vi "FilePath.vi"(9 "Data Root Path":path, 10 "File Type":enum16{"Thru", "NEXT", "FEXT"}(ring), 11 "Product Type":enum16{"QSFP28", "SFP28", "MiniSAS"}(ring)) -> (2 "File Path List":path[](array[path]), 3 "FileName List (not suffix)":string[](array[string]))   [LabVIEW 2011]
uses:
  <vilib>/Utility/file.llb/Read From Spreadsheet File (string).vi
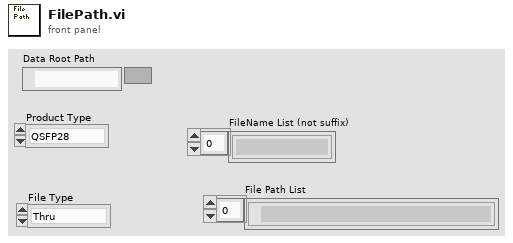
[diagram p1: front panel]
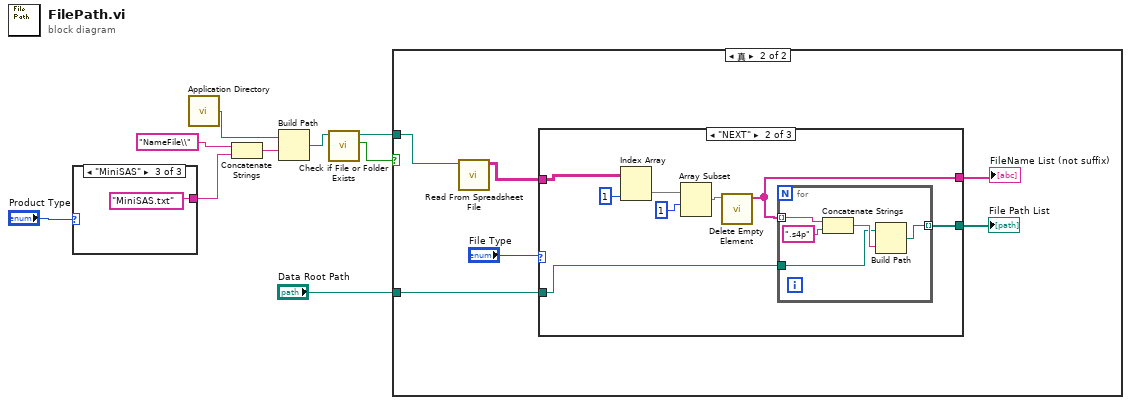
[diagram p0: block diagram]
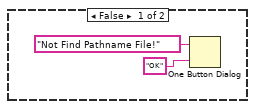
[diagram p2: hidden frame]
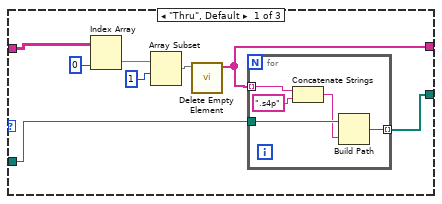
[diagram p3: hidden frame]
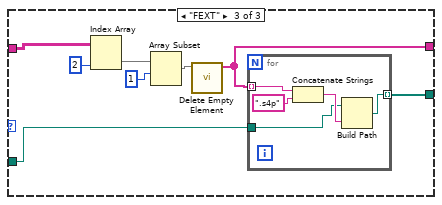
[diagram p4: hidden frame]
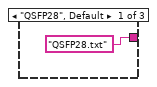
[diagram p5: hidden frame]
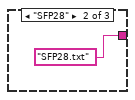
[diagram p6: hidden frame]
diagram:
  n1 = case shown="\"MiniSAS\"" "Product Type" {
    tunnel: ["QSFP28.txt" ("名称或相对路径") "SFP28.txt" ("名称或相对路径") "MiniSAS.txt" ("名称或相对路径")] -> w7
    frame "QSFP28", Default {
    }
    frame "SFP28" {
    }
    frame "MiniSAS" {
    }
  }
  n2 = call <vilib>:"Application Directory.vi"() -> ("Application Directory"=w8:path)
  n3 = Concatenate Strings("NameFile\\" ("字符串"), w7) -> (w5:string)
  n4 = Build Path(base path=w8, name or relative path=w5) -> (appended path=w4:path)
  n5 = call <vilib>:"Check if File or Folder Exists.vi"("path"=w4) -> ("file or folder exists?"=w2:bool, "dup path"=w3:path)  [unwired: 8 in, 1 out]
  n6 = case shown="真" w2 {
    tunnel: w3 -> [_ w17]
    tunnel: "Data Root Path" -> [_ w16]
    frame False {
      n7 = One Button Dialog(message="Not Find Pathname File!" ("消息"), button name ("OK")="OK" ("按钮名称（“确定”）")) -> ()  [unwired: 1 out]
    }
    frame True {
      n8 = call-poly <vilib>:"Read From Spreadsheet File.vi"("file path (dialog if empty)"=w17) -> ("all rows"=w19:string[][])  [unwired: 6 in, 4 out]
      n9 = case shown="\"NEXT\"" "File Type" {
        tunnel: w19 -> [w28 w41 w54]
        tunnel: [w23 w36 w49] -> w18
        tunnel: w16 -> [w22 w35 w48]
        tunnel: [w21 w34 w47] -> w15
        frame "Thru", Default {
          n10 = Index Array(array=w28, index (col)=0 ("禁用的索引 (列)")) -> (element=w26:string[])  [unwired: 1 in]
          n11 = Array Subset(array=w26, index=1 ("索引")) -> (w24:string[])  [unwired: 1 in]
          n12 = call "Delete Empty Element.vi"("input"=w24) -> ("output"=w23:string[])  [unwired: 10 in]
          n13 = for {
            tunnel: w23 -> [w33] mode=indexing
            tunnel: w22 -> [w31]
            tunnel: [w29] -> w21 mode=indexing
            n14 = Concatenate Strings(w33, ".s4p" ("字符串")) -> (w30:string)
            n15 = Build Path(base path=w31, name or relative path=w30) -> (appended path=w29:path)
          }
        }
        frame "NEXT" {
          n16 = Index Array(array=w41, index (col)=1 ("禁用的索引 (列)")) -> (element=w39:string[])  [unwired: 1 in]
          n17 = Array Subset(array=w39, index=1 ("索引")) -> (w37:string[])  [unwired: 1 in]
          n18 = call "Delete Empty Element.vi"("input"=w37) -> ("output"=w36:string[])  [unwired: 10 in]
          n19 = for {
            tunnel: w36 -> [w46] mode=indexing
            tunnel: w35 -> [w43]
            tunnel: [w42] -> w34 mode=indexing
            n20 = Concatenate Strings(w46, ".s4p" ("字符串")) -> (w44:string)
            n21 = Build Path(base path=w43, name or relative path=w44) -> (appended path=w42:path)
          }
        }
        frame "FEXT" {
          n22 = Index Array(array=w54, index (col)=2 ("禁用的索引 (列)")) -> (element=w52:string[])  [unwired: 1 in]
          n23 = Array Subset(array=w52, index=1 ("索引")) -> (w50:string[])  [unwired: 1 in]
          n24 = call "Delete Empty Element.vi"("input"=w50) -> ("output"=w49:string[])  [unwired: 10 in]
          n25 = for {
            tunnel: w49 -> [w59] mode=indexing
            tunnel: [w57] -> w47 mode=indexing
            tunnel: w48 -> [w55]
            n26 = Concatenate Strings(w59, ".s4p" ("字符串")) -> (w56:string)
            n27 = Build Path(base path=w55, name or relative path=w56) -> (appended path=w57:path)
          }
        }
      }
      "FileName List (not suffix)" <- w18
      "File Path List" <- w15
    }
  }
